vi "start.vi"(8 "error in (no error)":errorcluster, 11 "K2602 in":refnum<class "K2602.lvclass">) -> (0 "error out":errorcluster, 3 "K2602 out":refnum<class "K2602.lvclass">)   [LabVIEW 2009, in "Hardware.lvlib" / "Channels.lvlib" / "K2602.lvclass"]
doc: "Abstract Method\n\nStarts/Arms the AnalogOutput task. Normally the AnalogOutput device is configured to wait for a trigger signal, therefore, in this case the method Arms the device ready for recieving its trigger upon which it will start outputing immediately its data."
uses:
  K2602.lvclass
  K2602.lvclass/K2602.ctl
  <instrlib>/Keithley 2600 Series/Keithley 2600 Series.lvlib
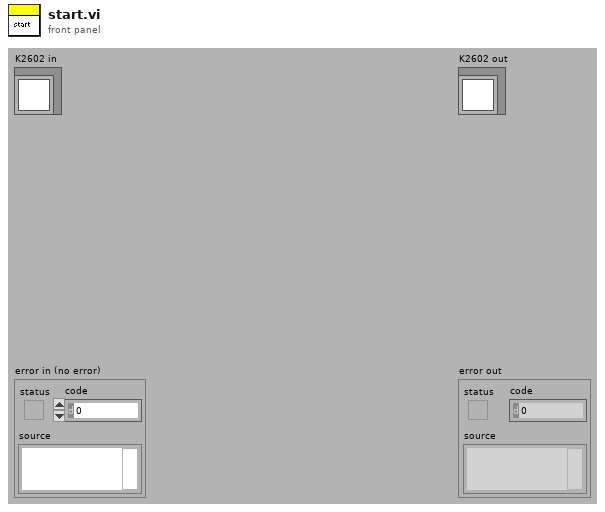
[diagram p1: front panel]
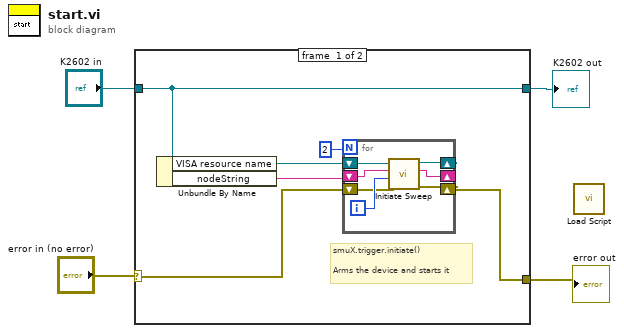
[diagram p0: block diagram]
diagram:
  n1 = case shown="No Error" "error in (no error)" {
    selector: "error in (no error)" -> [w6 w18]
    tunnel: [w10 w19] -> w3
    tunnel: "K2602 in" -> [w10 w19]
    tunnel: [w5 w18] -> w1
    frame #0 {
      # "smuX.trigger.initiate()\n\nArms the device and starts it"
      n2 = Unbundle By Name(w10) -> ("VISA resource name"=w8:refnum<visa-resource-name>, "nodeString"=w9:string)
      n3 = for {
        N: 2 -> [_]
        shift-right: [w12] -> _
        shift-left: w8 -> [w16]
        shift-right: [w11] -> _
        shift-left: w9 -> [w17]
        shift-right: [w13] -> w5
        shift-left: w6 -> [w14]
        i -> [w15]
        n4 = call <instrlib>:"Initiate Sweep.vi"("error in"=w14, "Channel (Channel A)"=w15, "Node In"=w17, "VISA resource name"=w16) -> ("error out"=w13:errorcluster, "Node Out"=w11:string, "VISA resource name out"=w12:refnum<visa-resource-name>)  [unwired: 4 in, 1 out]
      }
    }
    frame #1 {
    }
  }
  "error out" <- w1
  "K2602 out" <- w3
  n5 = call <instrlib>:"Load Script.vi"() -> ()  [unwired: 9 in, 3 out]
